vi "FindColllisionPoints.vi"(4 "ignoreBall?":bool, 6 "enemy_robots":T1[](array[typedef]), 7 "our_robots":T1[](array[typedef]), 8 "Robot in":T1={"id"=0, "function"=enum."Attacker", "x"=0.0, "y"=0.0, "orientation"=0.0, "v_tangent"=0.0, "v_normal"=0.0, "v_ang"=0.0, "kick_x"=0.0, "kick_z"=0.0, "dribble"=FALSE, "Timestamp"=timestamp(0 s since 1904-01-01), "estimatives"={"est_v_tangent"=0.0, "est_v_normal"=0.0, "est_vx"=0.0, "est_vy"=0.0, "Pos Robot Est"=[]}, "dest_x_kick"=0.0, "dest_y_kick"=0.0, "Gap Coord"=[], "States"=enum."Pass", "Path "=[], "Path  Smooth"=[], "Dest"=[], "vx_desired"=0.0, "vy_desired"=0.0, "slowBehavior"=FALSE, "VSSStates"=enum."Pass"}, 9 "Goal":dbl[](array[numeric]), 10 "Initial State":dbl[](array[numeric]), 11 "ball":dbl[](array[numeric])) -> (2 "Collision Points":dbl[][](array[numeric]))   [LabVIEW 2023]
uses:
  Vision_class/Old vision/Controls/AI Robot.ctl
  Vision_class/Old vision/Controls/Functions Enum.ctl
  Vision_class/Old vision/Controls/AttackerStates.ctl
  Vision_class/Old vision/Controls/PathDests.ctl
  Vision_class/Old vision/Controls/PathDest.ctl
  Navigation/VSSNavigation/VSSAttackerStates.ctl
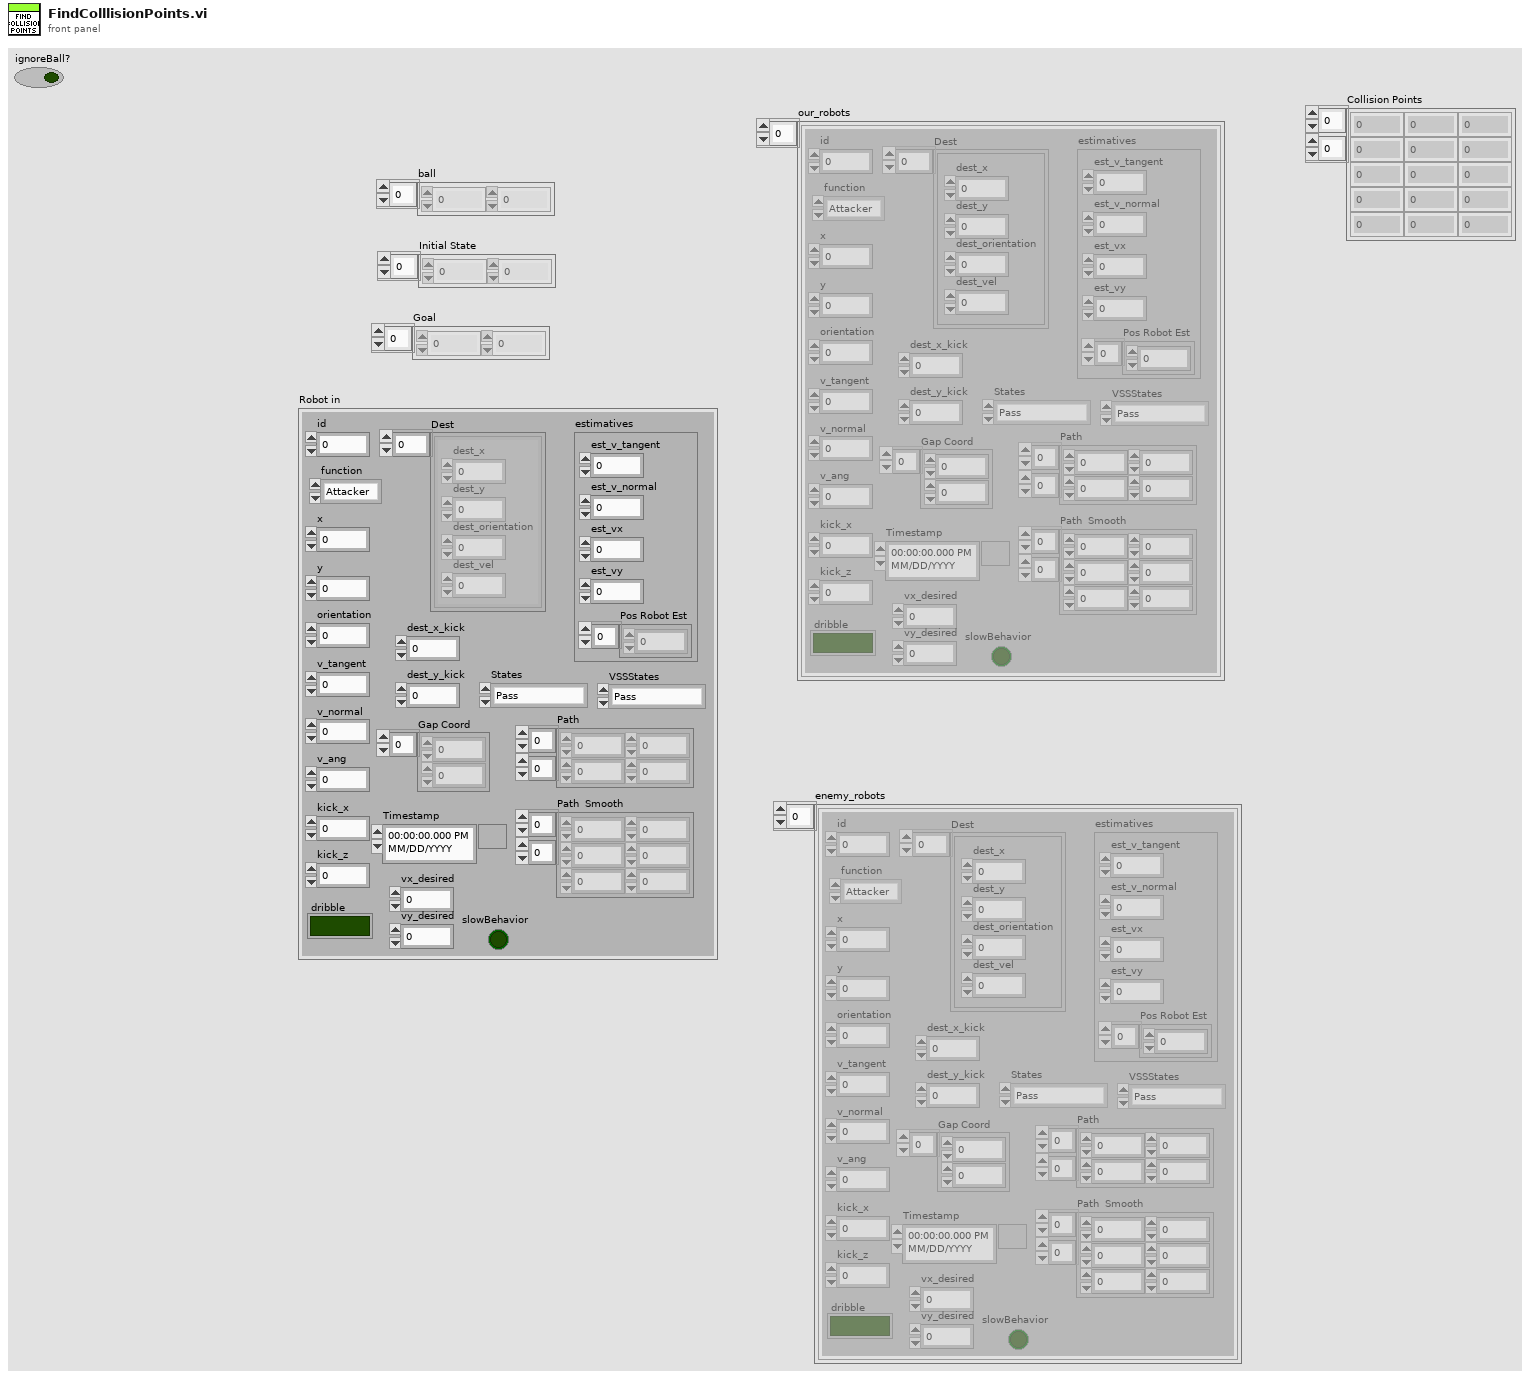
[diagram p1: front panel]
types:
  T1 = typedef "AI Robot.ctl" = cluster{"id":u32, "function":T2, "x":dbl, "y":dbl, "orientation":dbl, "v_tangent":dbl, "v_normal":dbl, "v_ang":dbl, "kick_x":dbl, "kick_z":dbl, "dribble":bool, "Timestamp":timestamp, "estimatives":cluster{"est_v_tangent":dbl, "est_v_normal":dbl, "est_vx":dbl, "est_vy":dbl, "Pos Robot Est":dbl[]}, "dest_x_kick":dbl, "dest_y_kick":dbl, "Gap Coord":dbl[], "States":T3, "Path ":dbl[][], "Path  Smooth":dbl[][], "Dest":T4, "vx_desired":dbl, "vy_desired":dbl, "slowBehavior":bool, "VSSStates":T6}
  T2 = typedef "Functions Enum.ctl" = enum16{"2nd Striker", "Attacker", "Goalie", "Defender", "Striker", "Goto 0", "Dummy", "Kicker", "ZigZag 0", "ZigZag 1", "ZigZag 2", "ZigZag 3", "ZigZag 4", "ZigZag 5", "ZigZag 6", "ZigZag 7", "ZigZag 8", ""}
  T3 = typedef "AttackerStates.ctl" = enum16{"Pass", "GoToTangent", "BallGetting", "GoToKick", ""}
  T4 = typedef "PathDests.ctl" = T5[]
  T5 = typedef "PathDest.ctl" = cluster{"dest_x":dbl, "dest_y":dbl, "dest_orientation":dbl, "dest_vel":dbl}
  T6 = typedef "VSSAttackerStates.ctl" = enum16{"Pass", "GoToTangent", "BallGetting", "GoToKick", "Rotate anti-clockwise", "Rotate Clockwise", ""}
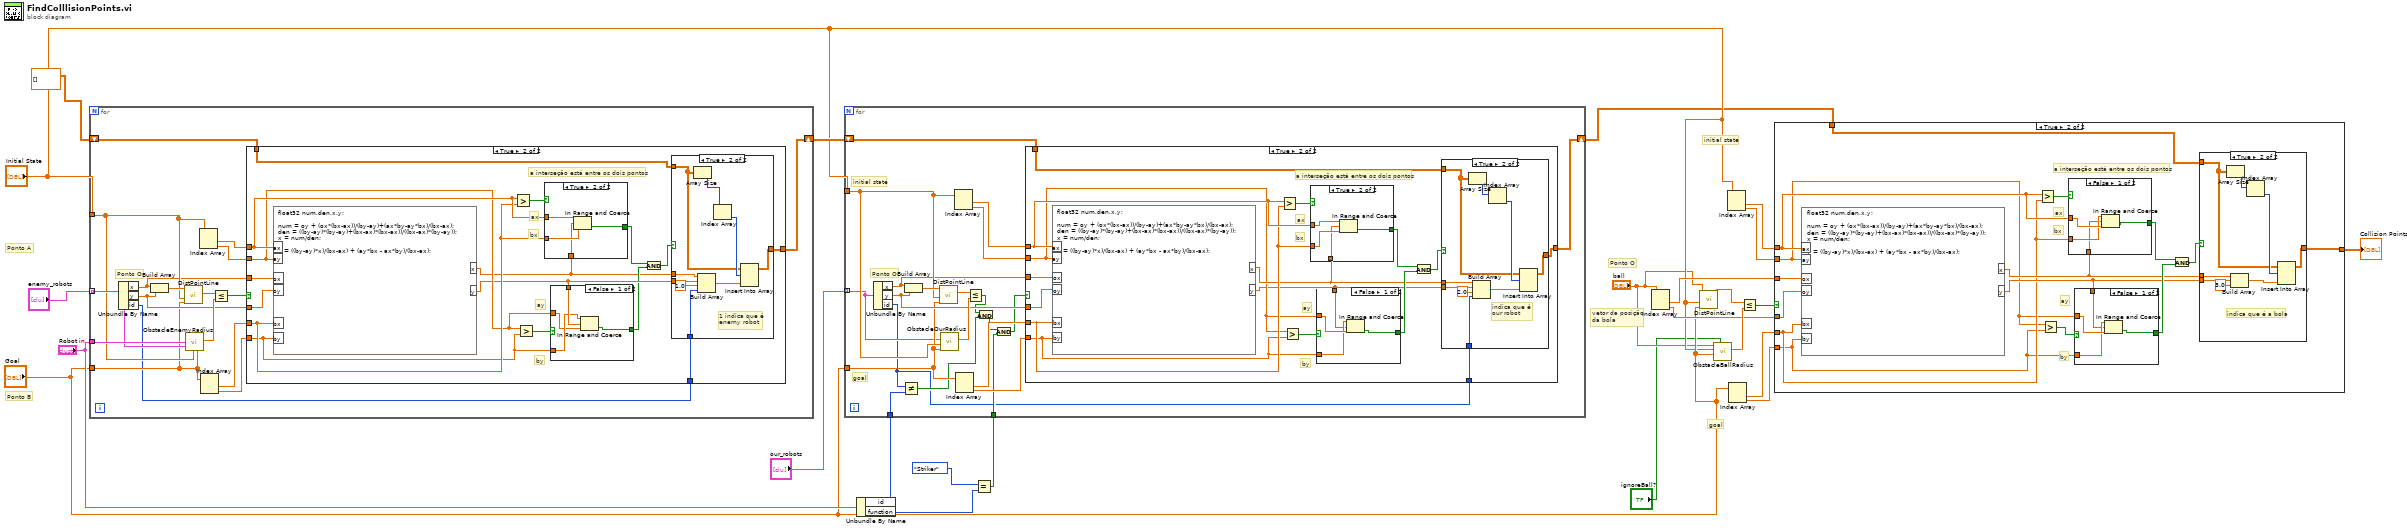
[diagram p0: block diagram]
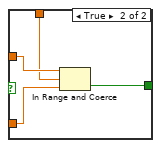
[diagram p4: hidden frame]
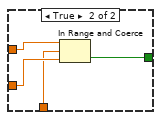
[diagram p5: hidden frame]
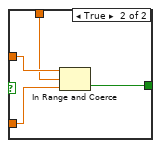
[diagram p8: hidden frame]
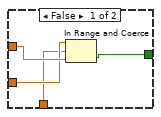
[diagram p9: hidden frame]
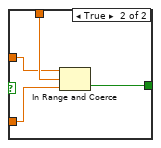
[diagram p12: hidden frame]
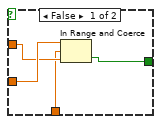
[diagram p13: hidden frame]
diagram:
  # "goal"
  # "initial state"
  # "Ponto O"
  # "vetor da posição\nda bola"
  # "Ponto B"
  # "Ponto A"
  n1 = for {
    tunnel: "enemy_robots" -> [w37] mode=indexing
    tunnel: "Initial State" -> [w33]
    tunnel: "Goal" -> [w28]
    tunnel: "Robot in" -> [w38]
    shift-right: [w34] -> w22
    shift-left: dbl[][] [] ("Path") -> [w35]
    # "Ponto O"
    n2 = Unbundle By Name(w37) -> ("x"=w30:dbl, "y"=w29:dbl, "id"=w25:u32)
    n3 = Build Array(w30, w29) -> (w41:dbl[])
    n4 = call "DistPointLine.vi"("P2"=w28, "P1"=w33, "Q"=w41) -> ("distance"=w40:dbl)  [unwired: 8 in]
    n5 = call "ObstacleEnemyRadius.vi"("Goal"=w28, "Initial State"=w33, "Robot enemy"=w37, "Robot in"=w38) -> ("obstacle enemy radius"=w39:dbl)  [unwired: 7 in]
    n6 = Index Array(array=w33) -> (element #1=w32:dbl, element #2=w31:dbl)  [unwired: 2 in]
    n7 = Index Array(array=w28) -> (element #1=w27:dbl, element #2=w26:dbl)  [unwired: 2 in]
    n8 = Less Or Equal?(x=w40, y=w39) -> (x <= y?=w36:bool)
    n9 = case shown="True" w36 {
      tunnel: w35 -> [w42 w56]
      tunnel: [w42 w55] -> w34
      tunnel: w32 -> [_ w53]
      tunnel: w31 -> [_ w50]
      tunnel: w30 -> [_ w58]
      tunnel: w29 -> [_ w57]
      tunnel: w27 -> [_ w52]
      tunnel: w26 -> [_ w49]
      tunnel: w25 -> [_ w43]
      frame False {
        # "obstáculo longe da trajetória"
      }
      frame True {
        # "a interseção está entre os dois pontos"
        # "by"
        # "ay"
        # "bx"
        # "ax"
        n10 = formula code="float32 num,den,x,y;\n\nnum = oy + (ox*(bx-ax))/(by-ay)+(ax*by-ay*bx)/(bx-ax);\nden = ((by-ay)*(by-ay)+(bx-ax)*(bx-ax))/((bx-ax)*(by-ay));\nx = num/den;\n\ny = ((by-ay)*x)/(bx-ax) + (ay*bx - ax*by)/(bx-ax);"("ax"=w53, "ay"=w50, "ox"=w58, "oy"=w57, "bx"=w52, "by"=w49) -> ("x"=w45:sgl, "y"=w48:sgl)
        n11 = Greater?(x=w53, y=w52) -> (0:w54:bool)
        n12 = Greater?(x=w50, y=w49) -> (0:w51:bool)
        n13 = case shown="True" w54 {
          tunnel: w53 -> [w79 w84]
          tunnel: w52 -> [w80 w83]
          tunnel: [w78 w82] -> w47
          tunnel: w45 -> [w77 w81]
          frame False {
            n14 = In Range and Coerce(upper limit=w80, x=w77, lower limit=w79) -> (In Range?=w78:bool)  [unwired: 1 out]
          }
          frame True {
            n15 = In Range and Coerce(upper limit=w84, x=w81, lower limit=w83) -> (In Range?=w82:bool)  [unwired: 1 out]
          }
        }
        n16 = case shown="False" w51 {
          tunnel: [w72 w76] -> w46
          tunnel: w50 -> [w69 w74]
          tunnel: w49 -> [w70 w73]
          tunnel: w48 -> [w71 w75]
          frame False {
            n17 = In Range and Coerce(upper limit=w70, x=w71, lower limit=w69) -> (In Range?=w72:bool)  [unwired: 1 out]
          }
          frame True {
            n18 = In Range and Coerce(upper limit=w74, x=w75, lower limit=w73) -> (In Range?=w76:bool)  [unwired: 1 out]
          }
        }
        n19 = And(x=w47, y=w46) -> (x .and. y?=w44:bool)
        n20 = case shown="True" w44 {
          tunnel: w56 -> [w59 w65]
          tunnel: [w59 w64] -> w55
          tunnel: w48 -> [_ w63]
          tunnel: w45 -> [_ w62]
          tunnel: w43 -> [_ w60]
          frame False {
          }
          frame True {
            # "1 indica que é\nenemy robot"
            n21 = Array Size(array=w65) -> (size(s)=w68:i32[])
            n22 = Build Array(w62, w63, sgl 1.0 ("element"), w60) -> (w66:sgl[])
            n23 = Index Array(array=w68) -> (element=w67:i32)  [unwired: 1 in]
            n24 = Insert Into Array(array=w65, index (row)=w67, new element=w66) -> (w64:dbl[][])  [unwired: 1 in]
          }
        }
      }
    }
  }
  n25 = Unbundle By Name("Robot in") -> ("id"=w19:u32, "function"=w4:T2)
  n26 = Equal?(x=Functions_Enum."Striker", y=w4) -> (x = y?=w2:bool)
  n27 = for {
    tunnel: "our_robots" -> [w92] mode=indexing
    tunnel: "Initial State" -> [w100]
    tunnel: "Goal" -> [w95]
    shift-right: [w101] -> w6
    shift-left: w22 -> [w102]
    tunnel: w19 -> [w91]
    tunnel: w2 -> [w87]
    # "goal"
    # "initial state"
    # "Ponto O"
    n28 = Unbundle By Name(w92) -> ("x"=w97:dbl, "y"=w96:dbl, "id"=w85:u32)
    n29 = Not Equal?(x=w85, y=w91) -> (x != y?=w89:bool)
    n30 = Build Array(w97, w96) -> (w105:dbl[])
    n31 = call "DistPointLine.vi"("P2"=w95, "P1"=w100, "Q"=w105) -> ("distance"=w104:dbl)  [unwired: 8 in]
    n32 = call "ObstacleOurRadius.vi"("Goal"=w95, "Initial State"=w100, "other robot"=w92) -> ("obstacle enemy radius"=w103:dbl)  [unwired: 8 in]
    n33 = Index Array(array=w100) -> (element #1=w99:dbl, element #2=w98:dbl)  [unwired: 2 in]
    n34 = Index Array(array=w95) -> (element #1=w94:dbl, element #2=w93:dbl)  [unwired: 2 in]
    n35 = Less Or Equal?(x=w104, y=w103) -> (x <= y?=w90:bool)
    n36 = And(x=w90, y=w89) -> (x .and. y?=w88:bool)
    n37 = And(x=w88, y=w87) -> (x .and. y?=w86:bool)
    n38 = case shown="True" w86 {
      tunnel: w102 -> [w106 w120]
      tunnel: [w106 w119] -> w101
      tunnel: w99 -> [_ w114]
      tunnel: w98 -> [_ w111]
      tunnel: w97 -> [_ w122]
      tunnel: w96 -> [_ w121]
      tunnel: w94 -> [_ w113]
      tunnel: w93 -> [_ w110]
      tunnel: w85 -> [_ w107]
      frame False {
        # "obstáculo longe da trajetória"
      }
      frame True {
        # "a interseção está entre os dois pontos"
        # "by"
        # "ay"
        # "bx"
        # "ax"
        n39 = formula code="float32 num,den,x,y;\n\nnum = oy + (ox*(bx-ax))/(by-ay)+(ax*by-ay*bx)/(bx-ax);\nden = ((by-ay)*(by-ay)+(bx-ax)*(bx-ax))/((bx-ax)*(by-ay));\nx = num/den;\n\ny = ((by-ay)*x)/(bx-ax) + (ay*bx - ax*by)/(bx-ax);"("ax"=w114, "ay"=w111, "ox"=w122, "oy"=w121, "bx"=w113, "by"=w110) -> ("x"=w112:sgl, "y"=w109:sgl)
        n40 = Greater?(x=w114, y=w113) -> (0:w118:bool)
        n41 = Greater?(x=w111, y=w110) -> (0:w117:bool)
        n42 = case shown="True" w118 {
          tunnel: [w144 w148] -> w116
          tunnel: w114 -> [w143 w147]
          tunnel: w113 -> [w142 w146]
          tunnel: w112 -> [w141 w145]
          frame False {
            n43 = In Range and Coerce(upper limit=w142, x=w141, lower limit=w143) -> (In Range?=w144:bool)  [unwired: 1 out]
          }
          frame True {
            n44 = In Range and Coerce(upper limit=w147, x=w145, lower limit=w146) -> (In Range?=w148:bool)  [unwired: 1 out]
          }
        }
        n45 = case shown="False" w117 {
          tunnel: [w136 w140] -> w115
          tunnel: w111 -> [w135 w139]
          tunnel: w110 -> [w134 w138]
          tunnel: w109 -> [w133 w137]
          frame False {
            n46 = In Range and Coerce(upper limit=w134, x=w133, lower limit=w135) -> (In Range?=w136:bool)  [unwired: 1 out]
          }
          frame True {
            n47 = In Range and Coerce(upper limit=w139, x=w137, lower limit=w138) -> (In Range?=w140:bool)  [unwired: 1 out]
          }
        }
        n48 = And(x=w116, y=w115) -> (x .and. y?=w108:bool)
        n49 = case shown="True" w108 {
          tunnel: w120 -> [w123 w129]
          tunnel: [w123 w128] -> w119
          tunnel: w112 -> [_ w127]
          tunnel: w109 -> [_ w126]
          tunnel: w107 -> [_ w124]
          frame False {
          }
          frame True {
            # "indica que é \nour robot"
            n50 = Array Size(array=w129) -> (size(s)=w132:i32[])
            n51 = Build Array(w127, w126, sgl 2.0 ("element"), w124) -> (w130:sgl[])
            n52 = Index Array(array=w132) -> (element=w131:i32)  [unwired: 1 in]
            n53 = Insert Into Array(array=w129, index (row)=w131, new element=w130) -> (w128:dbl[][])  [unwired: 1 in]
          }
        }
      }
    }
  }
  n54 = Index Array(array="ball") -> (element #1=w11:dbl, element #2=w10:dbl)  [unwired: 2 in]
  n55 = call "DistPointLine.vi"("P2"="Goal", "P1"="Initial State", "Q"="ball") -> ("distance"=w18:dbl)  [unwired: 8 in]
  n56 = call "ObstacleBallRadius.vi"("ignoreBall?"="ignoreBall?", "Goal"="Goal", "Initial State"="Initial State", "ball"="ball") -> ("obstacle enemy radius"=w17:dbl)  [unwired: 7 in]
  n57 = Index Array(array="Initial State") -> (element #1=w15:dbl, element #2=w14:dbl)  [unwired: 2 in]
  n58 = Index Array(array="Goal") -> (element #1=w13:dbl, element #2=w12:dbl)  [unwired: 2 in]
  n59 = Less Or Equal?(x=w18, y=w17) -> (x <= y?=w16:bool)
  n60 = case shown="True" w16 {
    tunnel: [w149 w154] -> w5
    tunnel: w15 -> [_ w153]
    tunnel: w14 -> [_ w150]
    tunnel: w11 -> [_ w164]
    tunnel: w10 -> [_ w163]
    tunnel: w13 -> [_ w152]
    tunnel: w12 -> [_ w151]
    tunnel: w6 -> [w149 w155]
    frame False {
      # "obstáculo longe da trajetória"
    }
    frame True {
      # "a interseção está entre os dois pontos"
      # "by"
      # "ay"
      # "bx"
      # "ax"
      n61 = formula code="float32 num,den,x,y;\n\nnum = oy + (ox*(bx-ax))/(by-ay)+(ax*by-ay*bx)/(bx-ax);\nden = ((by-ay)*(by-ay)+(bx-ax)*(bx-ax))/((bx-ax)*(by-ay));\nx = num/den;\n\ny = ((by-ay)*x)/(bx-ax) + (ay*bx - ax*by)/(bx-ax);"("ax"=w153, "ay"=w150, "ox"=w164, "oy"=w163, "bx"=w152, "by"=w151) -> ("x"=w157:sgl, "y"=w156:sgl)
      n62 = Greater?(x=w153, y=w152) -> (0:w162:bool)
      n63 = Greater?(x=w150, y=w151) -> (0:w161:bool)
      n64 = case shown="False" w162 {
        tunnel: [w185 w189] -> w160
        tunnel: w153 -> [w184 w188]
        tunnel: w152 -> [w183 w187]
        tunnel: w157 -> [w182 w186]
        frame False {
          n65 = In Range and Coerce(upper limit=w183, x=w182, lower limit=w184) -> (In Range?=w185:bool)  [unwired: 1 out]
        }
        frame True {
          n66 = In Range and Coerce(upper limit=w188, x=w186, lower limit=w187) -> (In Range?=w189:bool)  [unwired: 1 out]
        }
      }
      n67 = case shown="False" w161 {
        tunnel: [w177 w181] -> w159
        tunnel: w150 -> [w176 w180]
        tunnel: w151 -> [w175 w179]
        tunnel: w156 -> [w174 w178]
        frame False {
          n68 = In Range and Coerce(upper limit=w175, x=w174, lower limit=w176) -> (In Range?=w177:bool)  [unwired: 1 out]
        }
        frame True {
          n69 = In Range and Coerce(upper limit=w180, x=w178, lower limit=w179) -> (In Range?=w181:bool)  [unwired: 1 out]
        }
      }
      n70 = And(x=w160, y=w159) -> (x .and. y?=w158:bool)
      n71 = case shown="True" w158 {
        tunnel: w155 -> [w165 w170]
        tunnel: [w165 w169] -> w154
        tunnel: w157 -> [_ w168]
        tunnel: w156 -> [_ w167]
        frame False {
        }
        frame True {
          # "indica que é a bola"
          n72 = Array Size(array=w170) -> (size(s)=w173:i32[])
          n73 = Build Array(w168, w167, sgl 3.0 ("element")) -> (w171:sgl[])
          n74 = Index Array(array=w173) -> (element=w172:i32)  [unwired: 1 in]
          n75 = Insert Into Array(array=w170, index (row)=w172, new element=w171) -> (w169:dbl[][])  [unwired: 1 in]
        }
      }
    }
  }
  "Collision Points" <- w5
